vi "QCP_SetDblArr.vi"(6 "Add if New?":bool, 8 "error in":errorcluster, 9 "Values":dbl[](array[numeric]), 10 "Name":string, 11 "QCP_DevRef_In":T1) -> (0 "error out":errorcluster, 3 "QCP_DevRef_Out":T1)   [LabVIEW 2016]
uses:
  <userlib>/836-libraries/System/QCP_V2/QCPSupportCode/QCP_RefNum.ctl
  <userlib>/836-libraries/System/QCP_V2/QCPSupportCode/QCPData.ctl
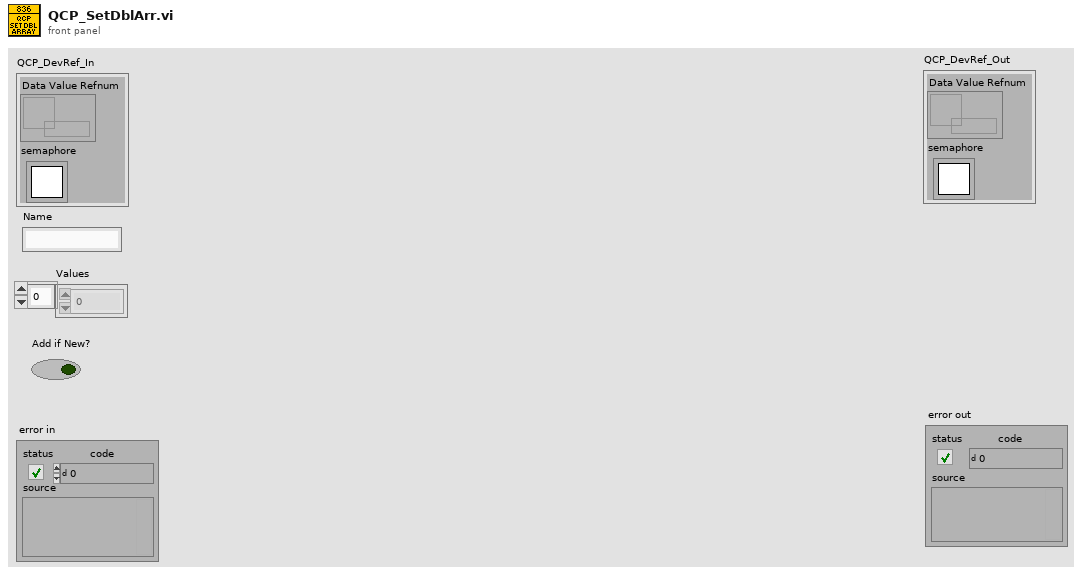
[diagram p1: front panel]
types:
  T1 = typedef "QCP_RefNum.ctl" = cluster{"Data Value Refnum":refnum<data-value>, "semaphore":T2}
  T2 = typedef "Semaphore RefNum" = refnum<k1>
  T3 = typedef "QCPData.ctl" = cluster{"Names":string[], "Values":cluster{"Array":dbl[]}[], "TuningMode?":bool}
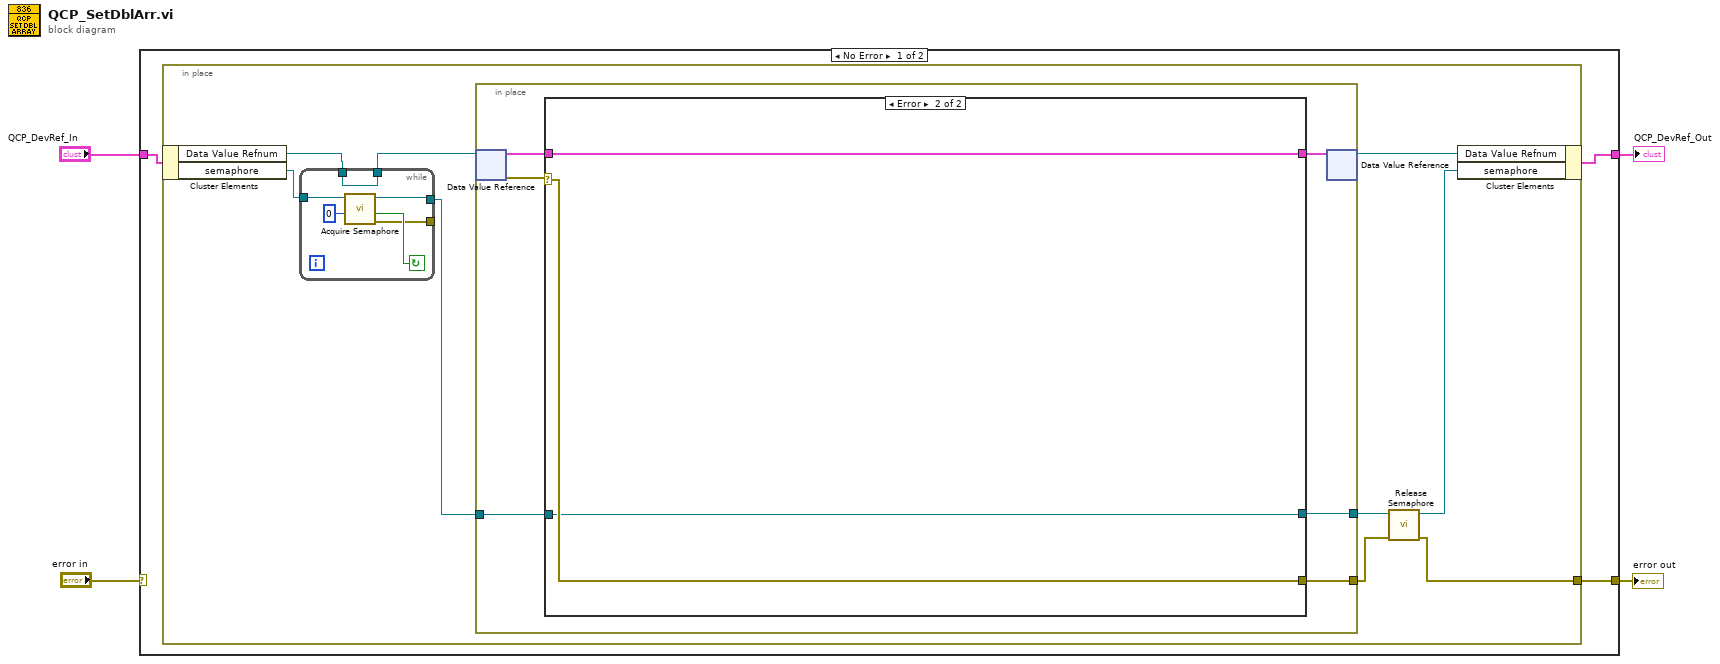
[diagram p0: block diagram]
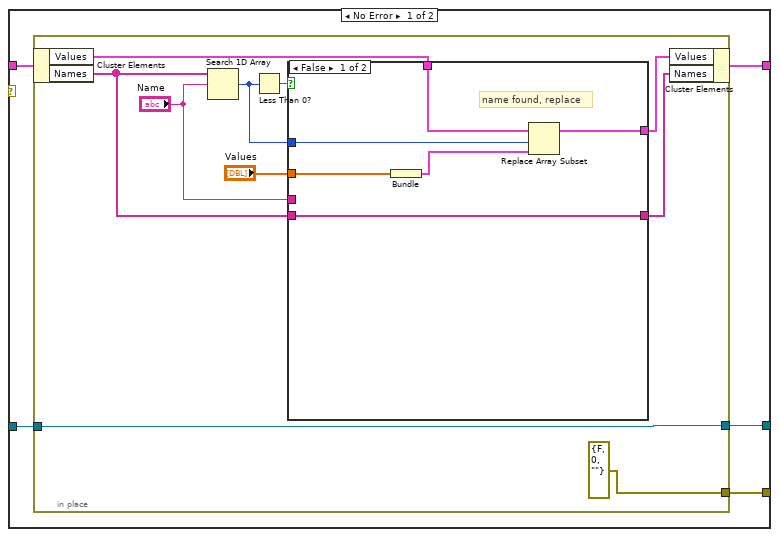
[diagram p2: hidden frame]
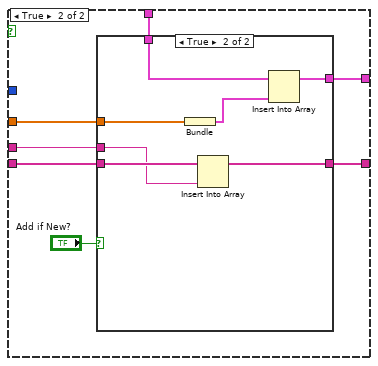
[diagram p3: hidden frame]
diagram:
  n1 = case shown="No Error" "error in" {
    selector: "error in" -> [_ w70]
    tunnel: [w5 w70] -> w3
    tunnel: "QCP_DevRef_In" -> [w7 w69]
    tunnel: [w6 w69] -> w1
    frame No Error {
      n2 = in-place {
        in-place-border: [w8] -> w5
        n3 = in-place-cluster #1(w7) -> ("Data Value Refnum"=w14:refnum<data-value>, "semaphore"=w15:T2)
        n4 = while {
          tunnel: [w21] -> _
          tunnel: [w20] -> w12
          tunnel: w15 -> [w19]
          tunnel: w14 -> [w18]
          tunnel: [w18] -> w13
          stop <- w22 continue-if-true
          n5 = call <vilib>:"Acquire Semaphore.vi"("ms timeout (-1)"=0, "semaphore"=w19) -> ("error out"=w21:errorcluster, "timed out"=w22:bool, "semaphore out"=w20:T2)  [unwired: 3 in]
        }
        n6 = in-place {
          in-place-border: [w27] -> w9
          in-place-border: w12 -> [w24]
          in-place-border: [w23] -> w10
          n7 = in-place-dvr #2(w13) -> (w26:T3, w28:errorcluster)
          n8 = case shown="Error" w28 {
            selector: w28 -> [_ w68]
            tunnel: [w31 w68] -> w27
            tunnel: w26 -> [w33 w67]
            tunnel: [w32 w67] -> w25
            tunnel: w24 -> [w30 w66]
            tunnel: [w29 w66] -> w23
            frame No Error {
              n9 = in-place {
                in-place-border: [errorcluster {"status"=FALSE, "code"=0, "source"=""} ("error constant")] -> w31
                in-place-border: [w34] -> w29
                in-place-border: w30 -> [w34]
                n10 = in-place-cluster #3(w33) -> ("Values"=w42:cluster{"Array":dbl[]}[], "Names"=w40:string[])
                n11 = Search 1D Array(1D array=w40, element="Name") -> (index of element=w41:i32)  [unwired: 1 in]
                n12 = Less Than 0?(x=w41) -> (x < 0?=w43:bool)
                n13 = case shown="False" w43 {
                  tunnel: w42 -> [w49 w54]
                  tunnel: w41 -> [w48 _]
                  tunnel: w40 -> [w44 w53]
                  tunnel: "Values" -> [w47 w50]
                  tunnel: [w45 w55] -> w39
                  tunnel: [w44 w52] -> w38
                  tunnel: "Name" -> [_ w51]
                  frame False {
                    # "name found, replace"
                    n14 = Bundle("Values"=w47) -> (w46:cluster{"Values":dbl[]})  [unwired: 1 in]
                    n15 = Replace Array Subset(array=w49, new element=w46, index=w48) -> (w45:cluster{"Array":dbl[]}[])
                  }
                  frame True {
                    n16 = case shown="True" "Add if New?" {
                      tunnel: [w58 w63] -> w55
                      tunnel: w54 -> [w58 w65]
                      tunnel: w53 -> [w57 w62]
                      tunnel: [w57 w60] -> w52
                      tunnel: w51 -> [_ w61]
                      tunnel: w50 -> [_ w59]
                      frame False {
                      }
                      frame True {
                        n17 = Bundle("Values"=w59) -> (w64:cluster{"Values":dbl[]})  [unwired: 1 in]
                        n18 = Insert Into Array(array=w62, new element=w61) -> (w60:string[])  [unwired: 1 in]
                        n19 = Insert Into Array(array=w65, new element=w64) -> (w63:cluster{"Array":dbl[]}[])  [unwired: 1 in]
                      }
                    }
                  }
                }
                n20 = in-place-cluster #3("Values"=w39, "Names"=w38) -> (w32:T3)
              }
            }
            frame Error {
            }
          }
          n21 = in-place-dvr #2(w25) -> (w16:refnum<data-value>)  [unwired: 1 out]
        }
        n22 = call <vilib>:"Release Semaphore.vi"("error in (no error)"=w9, "semaphore"=w10) -> ("error out"=w8:errorcluster, "semaphore out"=w11:T2)  [unwired: 4 in]
        n23 = in-place-cluster #1("Data Value Refnum"=w16, "semaphore"=w11) -> (w6:T1)
      }
    }
    frame Error {
    }
  }
  "QCP_DevRef_Out" <- w1
  "error out" <- w3
